vi "CRYCheck Channel Info.vi"(9 "Is Input?":bool, 10 "Channel No":u8, 11 "Channel Name":string) -> (0 "Channel Info":T1={"ID"=0, "Name"="", "Digital"=FALSE, "Input"=FALSE, "Device Name"="", "Hardware Ch ID"=0, "Vmax (V)"=0.0, "Latency (samples)"=0.0, "Sampling Rate (Hz)"=0, "Bit Depth"=0, "Anti-aliasing Factor (%fs)"=0.475, "DAQmx Channel"="", "term config"=-1, "Coupling"=-1, "IEPE en"=FALSE, "ASIOChannel Name"="", "Audio Driver"=0, "ASIOChannel Index"=0} {"Coupling" items=["Default"=-1, "RSE"=10083, "NRSE"=10078, "Differential"=10106, "Pseudodifferential"=12529]; "term config" items=["Default"=-1, "RSE"=10083, "NRSE"=10078, "Differential"=10106, "Pseudodifferential"=12529]; "Anti-aliasing Factor (%fs)" format="%.2f"}, 1 "ID":i32, 2 "Selected  No":u8, 3 "Is exist?":bool)   [LabVIEW 2013]
uses:
  Typedef Control/CRYHardware Channel Info.ctl
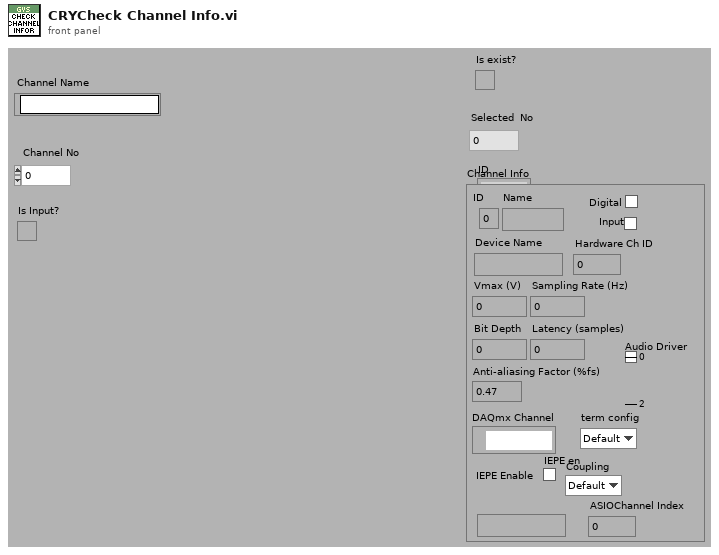
[diagram p1: front panel]
types:
  T1 = typedef "CRYHardware Channel Info.ctl" = cluster{"ID":i32, "Name":string, "Digital":bool, "Input":bool, "Device Name":string, "Hardware Ch ID":u8, "Vmax (V)":dbl, "Latency (samples)":dbl, "Sampling Rate (Hz)":u32, "Bit Depth":u32, "Anti-aliasing Factor (%fs)":sgl, "DAQmx Channel":tag, "term config":i32, "Coupling":i32, "IEPE en":bool, "ASIOChannel Name":string, "Audio Driver":u16, "ASIOChannel Index":u8}
  T2 = cluster{"StepName":string, "setup flattened":string}[]
  T3 = cluster{"StepName":string, "setup flattened":string}
  T4 = typedef "CRYHardware.ctl" = cluster{"Name":string, "Analog I/O":u16, "Digital I/O":u16, "Channels":u8, "Dig Dev ID":u8, "N ports":u8, "Interface":u32, "Dig I/O Ports":cluster{"port #":i16, "width":i16, "direction":i32}[], "Interf settings":cluster{"Type":u16, "COM Port":u8, "Baud rate":u32, "Data bits":u32, "Parity":u16, "Stop bits":u16, "Flow control":u16, "Dev ID IEEE":u8}[], "N interfs":i32, "udev SNs":i16[], "udev enable":bool, "Channel Array":T1[], "Cal sequence":string, "SelectedIn":u16, "SelectedOut":u16, "SelectedTab":u16, "State":bool, "Help":string, "Advanced":bool, "In Audio Driver":u16, "Out Audio Driver":u16}
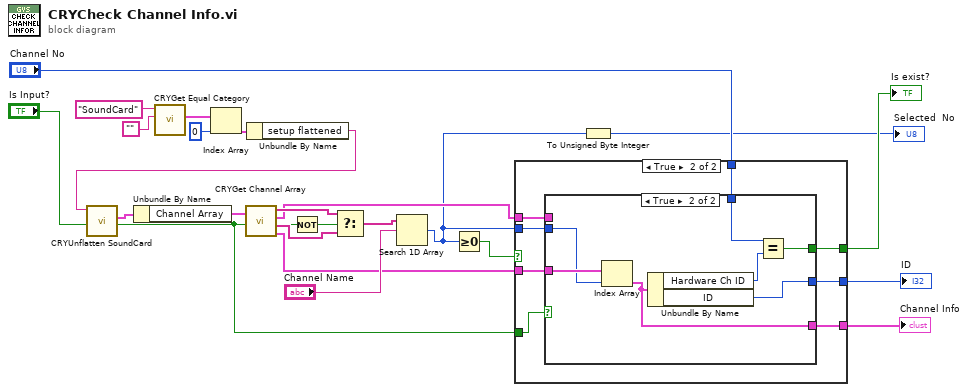
[diagram p0: block diagram]
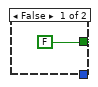
[diagram p2: hidden frame]
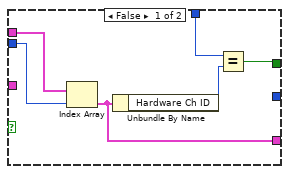
[diagram p3: hidden frame]
diagram:
  n1 = call "CRYGet Equal Category.vi"("Current StepName"="", "Find CategoryName"="SoundCard" ("CategoryName")) -> ("setup flattened Array out"=w23:T2)  [unwired: 9 out]
  n2 = Index Array(array=w23, index=0) -> (element=w20:T3)
  n3 = Unbundle By Name(w20) -> ("setup flattened"=w17:string)
  n4 = call "CRYUnflatten SoundCard.vi"("Flatten SoundCard"=w17) -> ("SoundCard"=w18:T4)  [unwired: 10 out]
  n5 = Unbundle By Name(w18) -> ("Channel Array"=w10:T1[])
  n6 = call "CRYGet Channel Array.vi"("Channel Array"=w10) -> ("I Channel Info Out"=w8:T1[], "I_Channel Name Out"=w14:string[], "O Channel Info Out"=w9:T1[], "O_Channel Name Out"=w15:string[])  [unwired: 7 out]
  n7 = Not(x="Is Input?") -> (.not. x?=w16:bool)
  n8 = Select(t=w15, s=w16, f=w14) -> (s? t:f=w13:string[])
  n9 = Search 1D Array(1D array=w13, element="Channel Name") -> (index of element=w4:i32)  [unwired: 1 out]
  n10 = Greater Or Equal To 0?(x=w4) -> (x >= 0?=w11:bool)
  n11 = case shown="True" w11 {
    tunnel: w9 -> [_ w29]
    tunnel: w8 -> [_ w31]
    tunnel: "Is Input?" -> [_ w32]
    tunnel: w4 -> [_ w30]
    tunnel: "Channel No" -> [_ w28]
    tunnel: [FALSE w27] -> w5
    tunnel: [_ w26] -> w2
    tunnel: [_ w25] -> w1
    frame False {
    }
    frame True {
      n12 = case shown="True" w32 {
        tunnel: w31 -> [_ w45]
        tunnel: w30 -> [w37 w44]
        tunnel: w29 -> [w38 _]
        tunnel: w28 -> [w36 w43]
        tunnel: [w34 w42] -> w27
        tunnel: [_ w40] -> w26
        tunnel: [w33 w39] -> w25
        frame False {
          n13 = Index Array(array=w38, index=w37) -> (element=w33:T1)
          n14 = Unbundle By Name(w33) -> ("Hardware Ch ID"=w35:u8)
          n15 = Equal?(x=w36, y=w35) -> (x = y?=w34:bool)
        }
        frame True {
          n16 = Index Array(array=w45, index=w44) -> (element=w39:T1)
          n17 = Unbundle By Name(w39) -> ("Hardware Ch ID"=w41:u8, "ID"=w40:i32)
          n18 = Equal?(x=w43, y=w41) -> (x = y?=w42:bool)
        }
      }
    }
  }
  "Is exist?" <- w5
  "ID" <- w2
  "Channel Info" <- w1
  n19 = To Unsigned Byte Integer(number=w4) -> (unsigned 8bit integer=→"Selected  No":u8)
